vi "dfd_Create Filter Coef from ZPK without Attributes.vi"(8 "error in (no error)":errorcluster, 9 "gain":dbl, 10 "poles":cdb[](array[numeric]), 11 "zeros":cdb[](array[numeric])) -> (0 "error out":errorcluster, 3 "filter coef out":T1)   [LabVIEW 2017, in "NI_DigFilterLicensed.lvlib"]
uses:
  <vilib>/addons/Digital Filter Design/NI_DigFilterLicensed.lvlib
  <vilib>/addons/Digital Filter Design/_Objects.llb/DFD Filter Coef.ctl
  <vilib>/addons/Digital Filter Design/_Objects.llb/DFD Filter Structure Type Selector.ctl
  <vilib>/Analysis/polynomials.llb/Create Polynomial From Roots (CDB).vi
  <vilib>/addons/Digital Filter Design/_Misc.llb/dfd_Error Handlers (Single).vi
  <vilib>/Analysis/NI_AALPro.lvlib
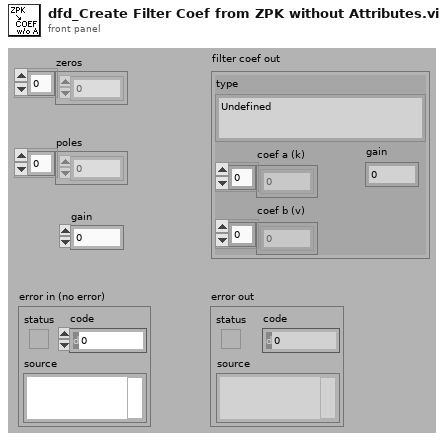
[diagram p1: front panel]
types:
  T1 = typedef "NI_DigFilterLicensed.lvlib/DFD Filter Coef.ctl" = cluster{"type":T2, "gain":dbl, "coef a (k)":dbl[], "coef b (v)":dbl[]}
  T2 = typedef "NI_DigFilterLicensed.lvlib/DFD Filter Structure Type Selector.ctl" = enum16{"Undefined", "FIR Direct Form", "FIR Direct Form Transposed", "FIR Symmetric", "FIR Antisymmetric", "IIR Direct Form I", "IIR Direct Form I Transposed", "IIR Direct Form II", "IIR Direct Form II Transposed", "IIR Cascaded Second Order Sections Form I", "IIR Cascaded Second Order Sections Form I Transposed", "IIR Cascaded Second Order Sections Form II", "IIR Cascaded Second Order Sections Form II Transposed", "Lattice Allpass (basic sections)", "Lattice Allpass (one multiplier sections)", "Lattice Allpass (normalized sections)", "Lattice AR (basic sections)", "Lattice AR (one multiplier sections)", "Lattice AR (normalized sections)", "Lattice MA (minimum phase)", "Lattice MA (maximum phase)", "Lattice ARMA (basic sections)", "Lattice ARMA (one multiplier sections)", "Lattice ARMA (normalized sections)"}
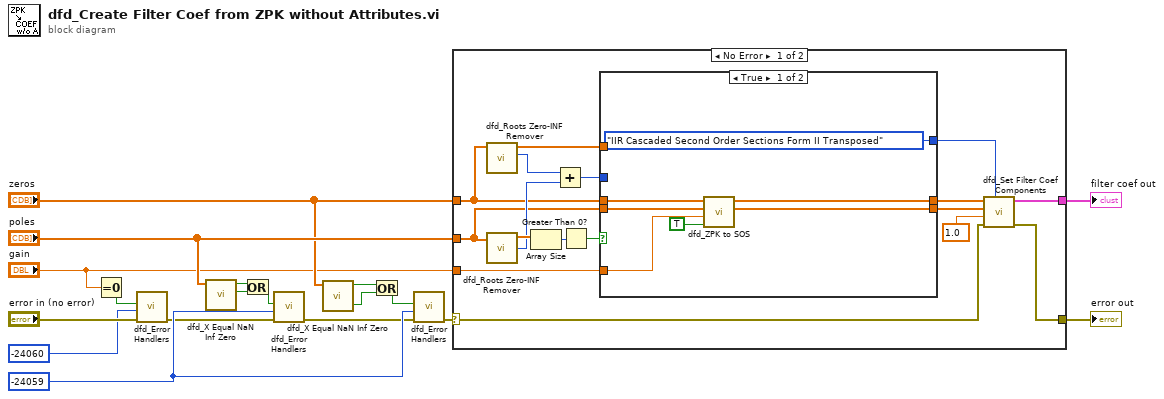
[diagram p0: block diagram]
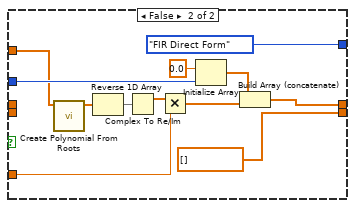
[diagram p2: hidden frame]
diagram:
  w13 = -24059 ("ERR_ZERO_POLE_INVALID")
  n1 = Equal To 0?(x="gain") -> (x = 0?=w4:bool)
  n2 = call-poly <vilib>:"dfd_Error Handlers.vi"("error in (no error)"="error in (no error)", "error code"=-24060 ("ERR_GAIN_NOT_ZERO"), "condition failed?"=w4) -> ("error out"=w2:errorcluster)  [unwired: 8 out]
  n3 = call <vilib>:"dfd_X Equal NaN Inf Zero.vi"("roots"="poles") -> ("contain Inf ?"=w10:bool, "contain NaN ?"=w14:bool)  [unwired: 9 out]
  n4 = Or(x=w14, y=w10) -> (x .or. y?=w11:bool)
  n5 = call-poly <vilib>:"dfd_Error Handlers.vi"("error in (no error)"=w2, "error code"=w13, "condition failed?"=w11) -> ("error out"=w12:errorcluster)  [unwired: 8 out]
  n6 = call <vilib>:"dfd_X Equal NaN Inf Zero.vi"("roots"="zeros") -> ("contain zero ?"=w7:bool, "contain NaN ?"=w8:bool)  [unwired: 9 out]
  n7 = Or(x=w8, y=w7) -> (x .or. y?=w6:bool)
  n8 = call-poly <vilib>:"dfd_Error Handlers.vi"("error in (no error)"=w12, "error code"=w13, "condition failed?"=w6) -> ("error out"=w16:errorcluster)  [unwired: 8 out]
  n9 = case shown="No Error" w16 {
    selector: w16 -> [w28 w55]
    tunnel: "gain" -> [w35 _]
    tunnel: "zeros" -> [w22 _]
    tunnel: [w27 w55] -> w18
    tunnel: [w26 _] -> w17
    tunnel: "poles" -> [w23 _]
    frame No Error {
      n10 = call <vilib>:"dfd_Roots Zero-INF Remover.vi"("roots"=w22) -> ("# zero root"=w19:i32, "new roots"=w21:cdb[])  [unwired: 9 out]
      n11 = call <vilib>:"dfd_Roots Zero-INF Remover.vi"("roots"=w23) -> ("# zero root"=w24:i32, "new roots"=w25:cdb[])  [unwired: 9 out]
      n12 = Array Size(array=w25) -> (size(s)=w33:i32)
      n13 = Add(x=w19, y=w24) -> (x+y=w20:i32)
      n14 = Greater Than 0?(x=w33) -> (x > 0?=w34:bool)
      n15 = case shown="True" w34 {
        tunnel: w22 -> [w41 _]
        tunnel: w35 -> [w40 w52]
        tunnel: [DFD_Filter_Structure_Type_Selector."IIR Cascaded Second Order Sections Form II Transposed" ("struct typ") DFD_Filter_Structure_Type_Selector."FIR Direct Form" ("struct typ")] -> w31
        tunnel: [w39 w47] -> w32
        tunnel: [w38 dbl[] [] ("coefficients a")] -> w30
        tunnel: w23 -> [w37 _]
        tunnel: w20 -> [_ w44]
        tunnel: w21 -> [_ w43]
        frame True {
          n16 = call <vilib>:"dfd_ZPK to SOS.vi"("UP?"=TRUE, "gain"=w40, "poles"=w37, "zeros"=w41) -> ("SOS reverse coefficients"=w38:dbl[], "SOS forward coefficients"=w39:dbl[])  [unwired: 6 out]
        }
        frame False {
          n17 = call-poly <vilib>:"Create Polynomial From Roots.vi"("Roots"=w43) -> ("P(x)"=w54:cdb[])  [unwired: 10 out]
          n18 = Reverse 1D Array(array=w54) -> (reversed array=w48:cdb[])
          n19 = Complex To Re/Im(x + iy=w48) -> (x=w53:dbl[])  [unwired: 1 out]
          n20 = Multiply(x=w53, y=w52) -> (x*y=w51:dbl[])
          n21 = Initialize Array(0.0 ("element"), w44) -> (w45:dbl[])
          n22 = Build Array (concatenate)(w45, w51) -> (w47:dbl[])
        }
      }
      n23 = call <vilib>:"dfd_Set Filter Coef Components.vi"("type"=w31, "error in (no error)"=w28, "gain"=1.0, "coef a (k)"=w30, "coef b (v)"=w32) -> ("error out"=w27:errorcluster, "filter coef"=w26:T1)  [unwired: 5 out]
    }
    frame Error {
    }
  }
  "error out" <- w18
  "filter coef out" <- w17
